vi "Read Test Sequences.vi"(8 "error in (no error)":errorcluster, 11 "CK in":refnum<class "CK.lvclass">) -> (0 "error out":errorcluster, 2 "Test Sequences":T2(array[cluster]), 3 "CK out":refnum<class "CK.lvclass">)   [LabVIEW 2020, in "CK.lvclass"]
uses:
  CK.lvclass
  Controls/Register to Write.ctl
  CK.lvclass/CK.ctl
  PIC-device/PIC-Device.lvclass
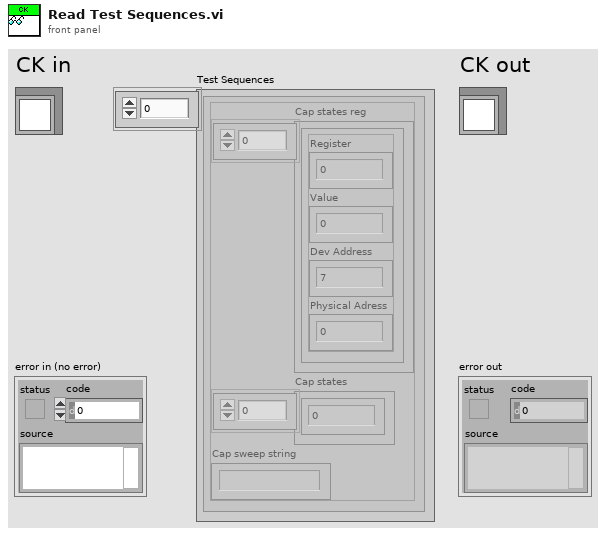
[diagram p1: front panel]
types:
  T1 = typedef "PIC-Device.lvclass/Register to Write.ctl" = cluster{"Register":u32, "Value":u32, "Dev Address":u32, "Physical Adress":u32}
  T2 = cluster{"Cap states reg":T1[], "Cap states":dbl[], "Cap sweep string":string}[]
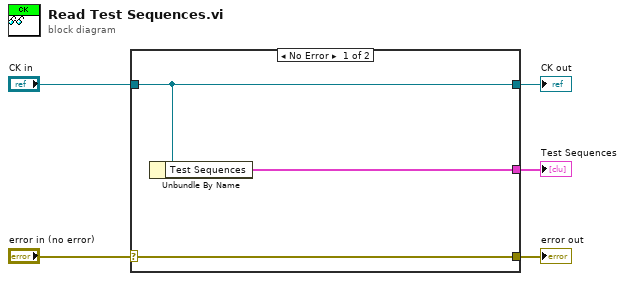
[diagram p0: block diagram]
diagram:
  n1 = case shown="No Error" "error in (no error)" {
    selector: "error in (no error)" -> [w8 w9]
    tunnel: [w8 w9] -> w4
    tunnel: [w7 w10] -> w2
    tunnel: "CK in" -> [w7 w10]
    tunnel: [w6 _] -> w1
    frame No Error {
      n2 = Unbundle By Name(w7) -> ("Test Sequences"=w6:T2)
    }
    frame Error {
    }
  }
  "error out" <- w4
  "CK out" <- w2
  "Test Sequences" <- w1
